vi "reprTextual.vi"(8 "error in (no error)":errorcluster, 11 "GenericMission in":refnum<class "GenericMission.lvclass">) -> (0 "error out":errorcluster, 2 "Description":string, 3 "GenericMission out":refnum<class "GenericMission.lvclass">)   [LabVIEW 2011, in "GenericMission.lvclass"]
uses:
  GenericMission.lvclass
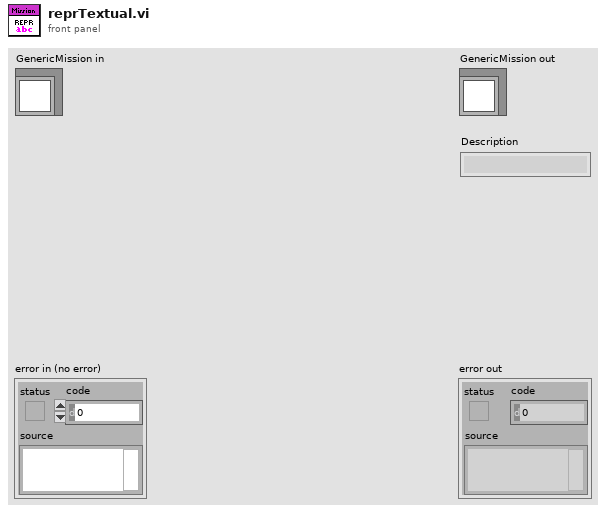
[diagram p1: front panel]
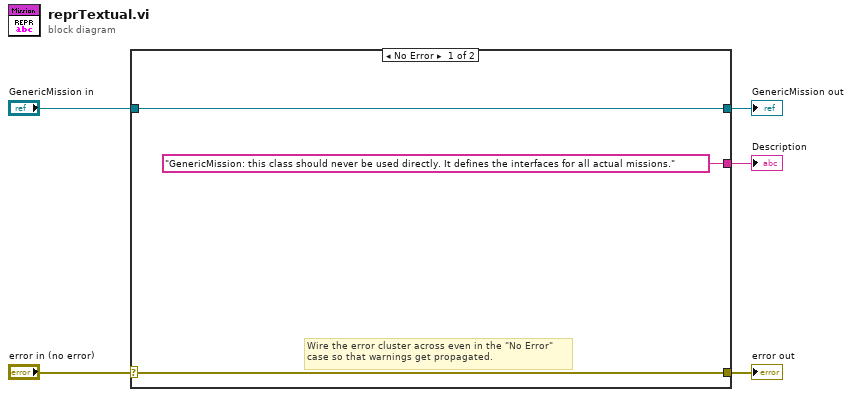
[diagram p0: block diagram]
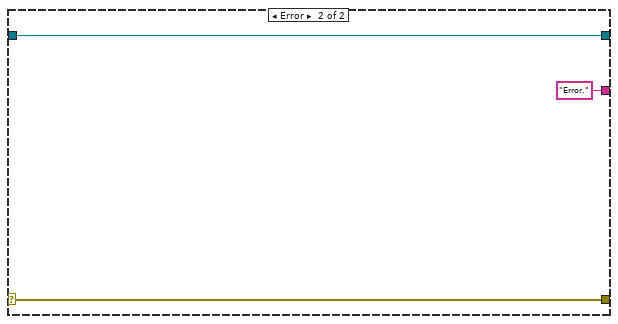
[diagram p2: hidden frame]
diagram:
  n1 = case shown="No Error" "error in (no error)" {
    selector: "error in (no error)" -> [w7 w11]
    tunnel: [w7 w11] -> w4
    tunnel: [w8 w10] -> w2
    tunnel: "GenericMission in" -> [w8 w10]
    tunnel: ["GenericMission: this class should never be used directly. It defines the interfaces for all actual missions." ("Description") "Error." ("Description")] -> w1
    frame No Error {
      # "Wire the error cluster across even in the \"No Error\"\ncase so that warnings get propagated."
    }
    frame Error {
    }
  }
  "error out" <- w4
  "GenericMission out" <- w2
  "Description" <- w1
